vi "绝缘电阻测试.vi"(8 "error in":errorcluster caption="错误输入", 10 "等待时间（毫秒）":u32=10000, 11 "Channel":u16=81 format="%.0x") -> (0 "error out":errorcluster caption="错误输出", 3 "绝缘电阻":u16)   [LabVIEW 2020]
uses:
  <userlib>/PCANBasic/ctl/TPCANMsgFD.ctl
  <userlib>/PCANBasic/PCANBasic.lvlib
panel:
  out "function return 2":u32 format="%.0x"
  out "function return 3":u32 format="%.0x"
  out "function return":u32 format="%.0x"
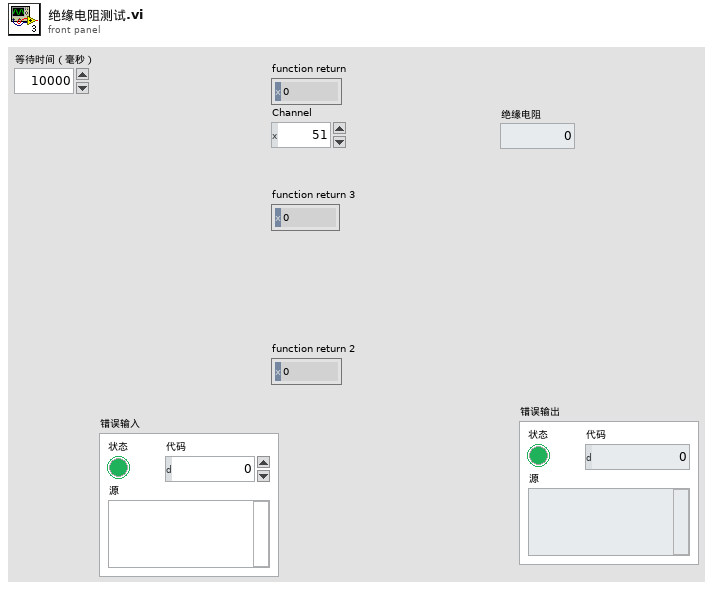
[diagram p1: front panel]
types:
  T1 = typedef "PCANBasic.lvlib/TPCANMsgFD.ctl" = cluster{"ID":u32, "MSGTYPE":u8, "DLC":u8, "DATA":cluster{"[0]":u8, "[1]":u8, "[2]":u8, "[3]":u8, "[4]":u8, "[5]":u8, "[6]":u8, "[7]":u8, "[8]":u8, "[9]":u8, "[10]":u8, "[11]":u8, "[12]":u8, "[13]":u8, "[14]":u8, "[15]":u8, "[16]":u8, "[17]":u8, "[18]":u8, "[19]":u8, "[20]":u8, "[21]":u8, "[22]":u8, "[23]":u8, "[24]":u8, "[25]":u8, "[26]":u8, "[27]":u8, "[28]":u8, "[29]":u8, "[30]":u8, "[31]":u8, "[32]":u8, "[33]":u8, "[34]":u8, "[35]":u8, "[36]":u8, "[37]":u8, "[38]":u8, "[39]":u8, "[40]":u8, "[41]":u8, "[42]":u8, "[43]":u8, "[44]":u8, "[45]":u8, "[46]":u8, "[47]":u8, "[48]":u8, "[49]":u8, "[50]":u8, "[51]":u8, "[52]":u8, "[53]":u8, "[54]":u8, "[55]":u8, "[56]":u8, "[57]":u8, "[58]":u8, "[59]":u8, "[60]":u8, "[61]":u8, "[62]":u8, "[63]":u8}}
  T2 = typedef "PCANBasic.lvlib/TPCANStatus.ctl" = u32
  T3 = cluster{"ID":u32, "MSGTYPE":u8, "DLC":u8, "DATA[0]":u8, "DATA[1]":u8, "DATA[2]":u8, "DATA[3]":u8, "DATA[4]":u8, "DATA[5]":u8, "DATA[6]":u8, "DATA[7]":u8, "DATA[8]":u8, "DATA[9]":u8, "DATA[10]":u8, "DATA[11]":u8, "DATA[12]":u8, "DATA[13]":u8, "DATA[14]":u8, "DATA[15]":u8, "DATA[16]":u8, "DATA[17]":u8, "DATA[18]":u8, "DATA[19]":u8, "DATA[20]":u8, "DATA[21]":u8, "DATA[22]":u8, "DATA[23]":u8, "DATA[24]":u8, "DATA[25]":u8, "DATA[26]":u8, "DATA[27]":u8, "DATA[28]":u8, "DATA[29]":u8, "DATA[30]":u8, "DATA[31]":u8, "DATA[32]":u8, "DATA[33]":u8, "DATA[34]":u8, "DATA[35]":u8, "DATA[36]":u8, "DATA[37]":u8, "DATA[38]":u8, "DATA[39]":u8, "DATA[40]":u8, "DATA[41]":u8, "DATA[42]":u8, "DATA[43]":u8, "DATA[44]":u8, "DATA[45]":u8, "DATA[46]":u8, "DATA[47]":u8, "DATA[48]":u8, "DATA[49]":u8, "DATA[50]":u8, "DATA[51]":u8, "DATA[52]":u8, "DATA[53]":u8, "DATA[54]":u8, "DATA[55]":u8, "DATA[56]":u8, "DATA[57]":u8, "DATA[58]":u8, "DATA[59]":u8, "DATA[60]":u8, "DATA[61]":u8, "DATA[62]":u8, "DATA[63]":u8}
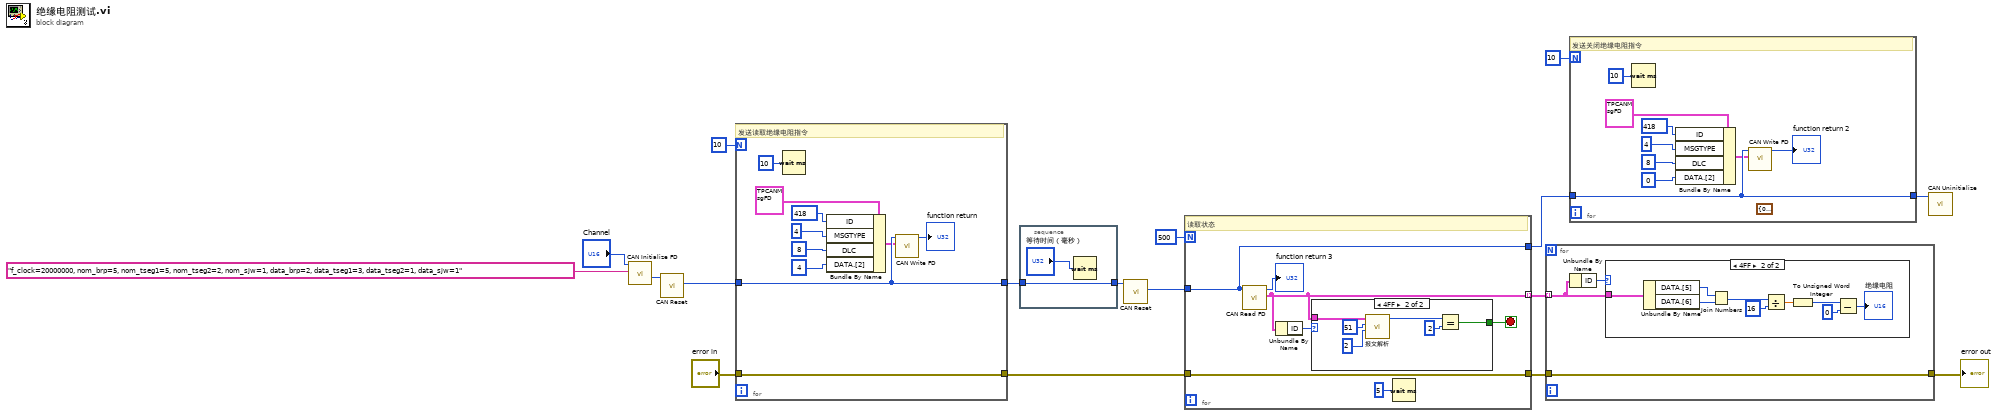
[diagram p0: block diagram]
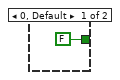
[diagram p3: hidden frame]
diagram:
  n1 = call <userlib>:"CAN Initialize FD.vi"("BitrateFD"="f_clock=20000000, nom_brp=5, nom_tseg1=5, nom_tseg2=2, nom_sjw=1, data_brp=2, data_tseg1=3, data_tseg2=1, data_sjw=1", "Channel"="Channel") -> ("Channel out"=w15:u16)  [unwired: 6 in, 3 out]
  n2 = call <userlib>:"CAN Reset.vi"("Channel in"=w15) -> ("Channel out"=w14:u16)  [unwired: 8 in, 2 out]
  n3 = for {
    N: 10 -> [_]
    tunnel: w14 -> [w25]
    tunnel: [w25] -> w12
    tunnel: "error in" -> [w19]
    tunnel: [w19] -> w3
    # "发送读取绝缘电阻指令"
    n4 = Wait (ms)(milliseconds to wait=u32 10 ("等待时间（毫秒）")) -> ()  [unwired: 1 out]
    n5 = Bundle By Name(cluster=T1 {"ID"=0, "MSGTYPE"=0, "DLC"=0, "DATA"={"[0]"=0, "[1]"=0, "[2]"=0, "[3]"=0, "[4]"=0, "[5]"=0, "[6]"=0, "[7]"=0, "[8]"=0, "[9]"=0, "[10]"=0, "[11]"=0, "[12]"=0, "[13]"=0, "[14]"=0, "[15]"=0, "[16]"=0, "[17]"=0, "[18]"=0, "[19]"=0, "[20]"=0, "[21]"=0, "[22]"=0, "[23]"=0, "[24]"=0, "[25]"=0, "[26]"=0, "[27]"=0, "[28]"=0, "[29]"=0, "[30]"=0, "[31]"=0, "[32]"=0, "[33]"=0, "[34]"=0, "[35]"=0, "[36]"=0, "[37]"=0, "[38]"=0, "[39]"=0, "[40]"=0, "[41]"=0, "[42]"=0, "[43]"=0, "[44]"=0, "[45]"=0, "[46]"=0, "[47]"=0, "[48]"=0, "[49]"=0, "[50]"=0, "[51]"=0, "[52]"=0, "[53]"=0, "[54]"=0, "[55]"=0, "[56]"=0, "[57]"=0, "[58]"=0, "[59]"=0, "[60]"=0, "[61]"=0, "[62]"=0, "[63]"=0}} ("MessageBuffer out"), "ID"=u32 418, "MSGTYPE"=u8 4, "DLC"=u8 8 ("ID"), "DATA.[2]"=u8 4 ("ID")) -> (w20:T1)
    n6 = call <userlib>:"CAN Write FD.vi"("MessageBuffer in"=w20, "Channel"=w25) -> ("TCANStatus"=→"function return":T2)  [unwired: 6 in, 3 out]
  }
  n7 = stacked-sequence {
    tunnel: w12 -> [w29]
    tunnel: [w29] -> w6
    frame #0 {
      n8 = Wait (ms)(milliseconds to wait="等待时间（毫秒）") -> ()  [unwired: 1 out]
    }
  }
  n9 = call <userlib>:"CAN Reset.vi"("Channel in"=w6) -> ("Channel out"=w5:u16)  [unwired: 8 in, 2 out]
  n10 = for {
    N: 500 -> [_]
    tunnel: w5 -> [w35]
    tunnel: [w32] -> w10 mode=indexing
    tunnel: [w35] -> w8
    tunnel: w3 -> [w30]
    tunnel: [w30] -> w2
    stop <- w31 stop-if-true
    # "读取状态"
    n11 = call <userlib>:"CAN Read FD.vi"("Channel"=w35) -> ("MessageBuffer out"=w32:T1, "TCANStatus"=→"function return 3":T2)  [unwired: 7 in, 2 out]
    n12 = Unbundle By Name(w32) -> ("ID"=w33:u32)
    n13 = case shown="4FF" w33 {
      tunnel: w32 -> [_ w41]
      tunnel: [FALSE w42] -> w31
      frame 0, Default {
      }
      frame 1279 {
        n14 = call "报文解析.vi"("长度"=2, "起始位"=51, "MessageBuffer in"=w41) -> ("数字"=w38:u32)  [unwired: 8 in]
        n15 = Equal?(x=w38, y=u8 2) -> (x = y?=w42:bool)
      }
    }
    n16 = Wait (ms)(milliseconds to wait=u32 5 ("等待时间（毫秒）")) -> ()  [unwired: 1 out]
  }
  n17 = for {
    tunnel: w10 -> [w45] mode=indexing
    tunnel: w2 -> [w44]
    tunnel: [w44] -> w1
    n18 = Unbundle By Name(w45) -> ("ID"=w46:u32)
    n19 = case shown="4FF" w46 {
      tunnel: w45 -> [_ w55]
      frame 0, Default {
      }
      frame 1279 {
        n20 = Unbundle By Name(w55) -> ("DATA.[5]"=w53:u8, "DATA.[6]"=w52:u8)
        n21 = Join Numbers(hi=w53, lo=w52) -> ((hi.lo)=w51:u16)
        n22 = Divide(x=w51, y=u8 16) -> (x/y=w49:dbl)
        n23 = To Unsigned Word Integer(number=w49) -> (unsigned 16bit integer=w48:u16)
        n24 = Subtract(x=w48, y=u16 0) -> (x-y=→"绝缘电阻":u16)
      }
    }
  }
  "error out" <- w1
  n25 = for {
    N: 10 -> [_]
    tunnel: w8 -> [w62]
    tunnel: [w62] -> w7
    (unwired) T3 {"ID"=0, "MSGTYPE"=0, "DLC"=0, "DATA[0]"=0, "DATA[1]"=0, "DATA[2]"=0, "DATA[3]"=0, "DATA[4]"=0, "DATA[5]"=0, "DATA[6]"=0, "DATA[7]"=0, "DATA[8]"=0, "DATA[9]"=0, "DATA[10]"=0, "DATA[11]"=0, "DATA[12]"=0, "DATA[13]"=0, "DATA[14]"=0, "DATA[15]"=0, "DATA[16]"=0, "DATA[17]"=0, "DATA[18]"=0, "DATA[19]"=0, "DATA[20]"=0, "DATA[21]"=0, "DATA[22]"=0, "DATA[23]"=0, "DATA[24]"=0, "DATA[25]"=0, "DATA[26]"=0, "DATA[27]"=0, "DATA[28]"=0, "DATA[29]"=0, "DATA[30]"=0, "DATA[31]"=0, "DATA[32]"=0, "DATA[33]"=0, "DATA[34]"=0, "DATA[35]"=0, "DATA[36]"=0, "DATA[37]"=0, "DATA[38]"=0, "DATA[39]"=0, "DATA[40]"=0, "DATA[41]"=0, "DATA[42]"=0, "DATA[43]"=0, "DATA[44]"=0, "DATA[45]"=0, "DATA[46]"=0, "DATA[47]"=0, "DATA[48]"=0, "DATA[49]"=0, "DATA[50]"=0, "DATA[51]"=0, "DATA[52]"=0, "DATA[53]"=0, "DATA[54]"=0, "DATA[55]"=0, "DATA[56]"=0, "DATA[57]"=0, "DATA[58]"=0, "DATA[59]"=0, "DATA[60]"=0, "DATA[61]"=0, "DATA[62]"=0, "DATA[63]"=0} ("MessageBuffer")
    # "发送关闭绝缘电阻指令"
    n26 = Wait (ms)(milliseconds to wait=u32 10 ("等待时间（毫秒）")) -> ()  [unwired: 1 out]
    n27 = Bundle By Name(cluster=T1 {"ID"=0, "MSGTYPE"=0, "DLC"=0, "DATA"={"[0]"=0, "[1]"=0, "[2]"=0, "[3]"=0, "[4]"=0, "[5]"=0, "[6]"=0, "[7]"=0, "[8]"=0, "[9]"=0, "[10]"=0, "[11]"=0, "[12]"=0, "[13]"=0, "[14]"=0, "[15]"=0, "[16]"=0, "[17]"=0, "[18]"=0, "[19]"=0, "[20]"=0, "[21]"=0, "[22]"=0, "[23]"=0, "[24]"=0, "[25]"=0, "[26]"=0, "[27]"=0, "[28]"=0, "[29]"=0, "[30]"=0, "[31]"=0, "[32]"=0, "[33]"=0, "[34]"=0, "[35]"=0, "[36]"=0, "[37]"=0, "[38]"=0, "[39]"=0, "[40]"=0, "[41]"=0, "[42]"=0, "[43]"=0, "[44]"=0, "[45]"=0, "[46]"=0, "[47]"=0, "[48]"=0, "[49]"=0, "[50]"=0, "[51]"=0, "[52]"=0, "[53]"=0, "[54]"=0, "[55]"=0, "[56]"=0, "[57]"=0, "[58]"=0, "[59]"=0, "[60]"=0, "[61]"=0, "[62]"=0, "[63]"=0}} ("MessageBuffer out"), "ID"=u32 418, "MSGTYPE"=u8 4, "DLC"=u8 8 ("ID"), "DATA.[2]"=u8 0 ("ID")) -> (w57:T1)
    n28 = call <userlib>:"CAN Write FD.vi"("MessageBuffer in"=w57, "Channel"=w62) -> ("TCANStatus"=→"function return 2":T2)  [unwired: 6 in, 3 out]
  }
  n29 = call <userlib>:"CAN Uninitialize.vi"("Channel"=w7) -> ()  [unwired: 9 in, 2 out]
